vi "Sweep.vi"(8 "error in (no error)":errorcluster, 11 "config":T1) -> (0 "error out":errorcluster, 3 "config out":T1)   [LabVIEW 2017, in "EmsaAcquisition.lvlib"]
uses:
  <vilib>/addons/InsightCM/Devices/Shared/Emsa/EmsaAcquisition/EmsaAcquisition.lvlib
  <vilib>/addons/InsightCM/Devices/Shared/Emsa/EmsaAcquisition/controls/config.ctl
  <vilib>/addons/InsightCM/Devices/Shared/Emsa/Emsa9770API/9770 API.lvclass
  <vilib>/addons/InsightCM/Devices/Shared/Emsa/EmsaAcquisition/controls/group.ctl
  <vilib>/addons/InsightCM/Devices/Shared/Emsa/EmsaAcquisition/controls/acqConfig.ctl
  <vilib>/addons/PointValueMap/subVIs/Point_Write_variant.vi
  <vilib>/addons/PointValueMap/PointValueMap.lvlib
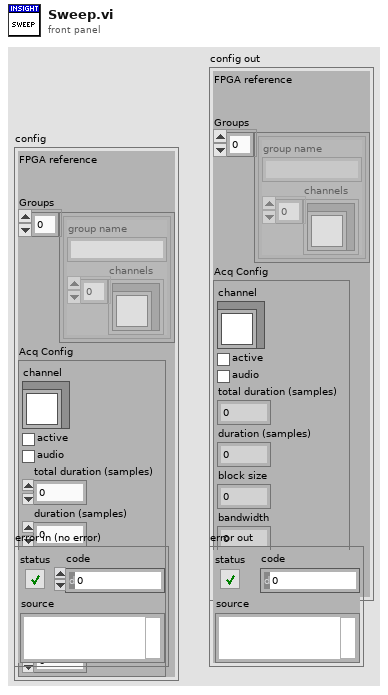
[diagram p1: front panel]
types:
  T1 = typedef "EmsaAcquisition.lvlib/config.ctl" = cluster{"FPGA reference":refnum<k20>, "Groups":T2[], "Acq Config":T3}
  T2 = typedef "EmsaAcquisition.lvlib/group.ctl" = cluster{"group name":string, "channels":refnum<class "9770 API.lvclass">[]}
  T3 = typedef "EmsaAcquisition.lvlib/acqConfig.ctl" = cluster{"channel":refnum<class "9770 API.lvclass">, "active":bool, "audio":bool, "total duration (samples)":i32, "duration (samples)":i32, "block size":i32, "bandwidth":dbl, "center frequency":dbl}
  T4 = typedef "PointValueMap.lvlib/PointMap.ctl" = refnum<data-value>
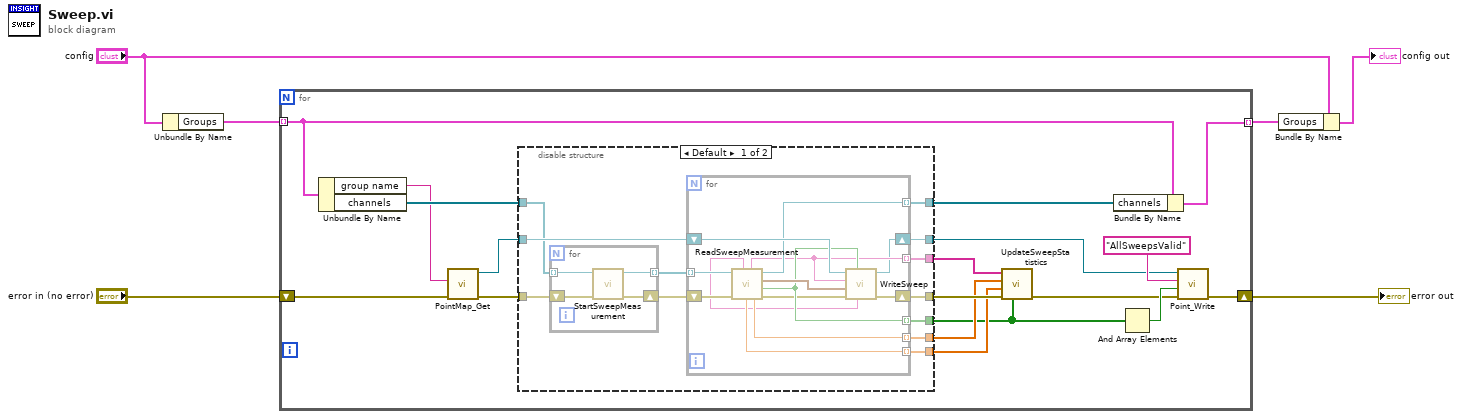
[diagram p0: block diagram]
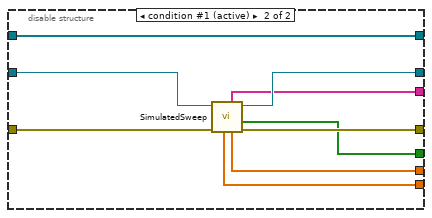
[diagram p2: hidden frame]
diagram:
  n1 = Unbundle By Name("config") -> ("Groups"=w3:T2[])
  n2 = for {
    shift-right: [w15] -> w2
    shift-left: "error in (no error)" -> [w21]
    tunnel: [w22] -> w5 mode=indexing
    tunnel: w3 -> [w13] mode=indexing
    n3 = Unbundle By Name(w13) -> ("group name"=w18:string, "channels"=w24:refnum<class "9770 API.lvclass">[])
    n4 = call <vilib>:"PointMap_Get.vi"("error in (no error)"=w21, "Name"=w18) -> ("error out"=w19:errorcluster, "Map Out"=w20:T4)  [unwired: 7 in, 1 out]
    n5 = disable-structure shown="Default" {
      disable-tunnel: w24 -> [w28 w62]
      disable-tunnel: [w36 w62] -> w23
      disable-tunnel: w20 -> [w35 w58]
      disable-tunnel: w19 -> [w29 w61]
      disable-tunnel: [w34 w57] -> w7
      disable-tunnel: [w25 w59] -> w16
      disable-tunnel: [w33 w60] -> w11
      disable-tunnel: [w32 w56] -> w10
      disable-tunnel: [w31 w54] -> w9
      disable-tunnel: [w30 w55] -> w8
      frame condition #0 {
        n6 = for {
          shift-right: [w39] -> w26
          shift-left: w29 -> [w40]
          tunnel: w28 -> [w38] mode=indexing
          tunnel: [w37] -> w27 mode=indexing
          n7 = call <vilib>:"StartSweepMeasurement.vi"("error in (no error)"=w40, "9770 API in"=w38) -> ("error out"=w39:errorcluster, "9770 API out"=w37:refnum<class "9770 API.lvclass">)  [unwired: 8 in]
        }
        n8 = for {
          tunnel: w27 -> [w50] mode=indexing
          shift-right: [w52] -> w33
          shift-left: w26 -> [w51]
          tunnel: [w49] -> w36 mode=indexing
          tunnel: [w47] -> w34 mode=indexing
          tunnel: [w42] -> w32 mode=indexing
          tunnel: [w45] -> w31 mode=indexing
          tunnel: [w44] -> w30 mode=indexing
          shift-right: [w41] -> w25
          shift-left: w35 -> [w53]
          n9 = call <vilib>:"ReadSweepMeasurement.vi"("error in (no error)"=w51, "9770 API in"=w50) -> ("error out"=w46:errorcluster, "sweep valid"=w47:bool, "sweep"=w48:cluster{"frequency":dbl, "amplitude":dbl}[], "9770 API out"=w49:refnum<class "9770 API.lvclass">, "sweep time (seconds)"=w45:dbl, "ChannelName"=w42:string, "current sweep frequency"=w44:dbl, "Units"=w43:string)  [unwired: 2 in]
          n10 = call <vilib>:"WriteSweep.vi"("unit"=w43, "sweep valid"=w47, "error in (no error)"=w46, "sweep"=w48, "channel"=w42, "map"=w53) -> ("error out"=w52:errorcluster, "map out"=w41:T4)  [unwired: 4 in]
        }
      }
      frame condition #1 (active) {
        n11 = call <vilib>:"SimulatedSweep.vi"("error in (no error)"=w61, "Map"=w58) -> ("error out"=w60:errorcluster, "Sweeps Valid"=w57:bool[], "map out"=w59:T4, "sweep times"=w54:dbl[], "channels"=w56:string[], "current sweep frequencies"=w55:dbl[])  [unwired: 4 in]
      }
    }
    n12 = call <vilib>:"UpdateSweepStatistics.vi"("sweep complete"=w7, "error in (no error)"=w11, "current sweep frequencies"=w8, "sweep times"=w9, "channels"=w10) -> ("error out"=w12:errorcluster)  [unwired: 6 in]
    n13 = Bundle By Name(cluster=w13, "channels"=w23) -> (w22:T2)
    n14 = And Array Elements(Boolean array=w7) -> (logical AND=w14:bool)
    n15 = call-poly <vilib>:"Point_Write.vi"("Error In"=w12, "Value"=w14, "Tag"="AllSweepsValid", "Map"=w16) -> ("Error Out"=w15:errorcluster)  [unwired: 6 in, 1 out]
  }
  "error out" <- w2
  n16 = Bundle By Name(cluster="config", "Groups"=w5) -> (→"config out":T1)
